vi "blink led.vi"() -> ()   [LabVIEW 2020]
panel:
  in  "stop":bool
  out "Boolean":bool
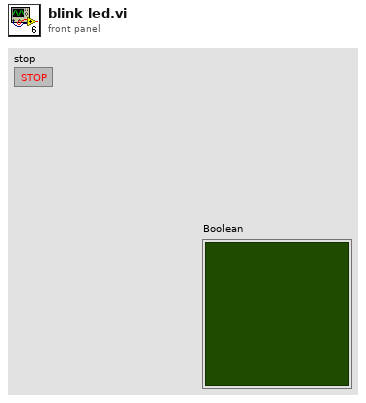
[diagram p1: front panel]
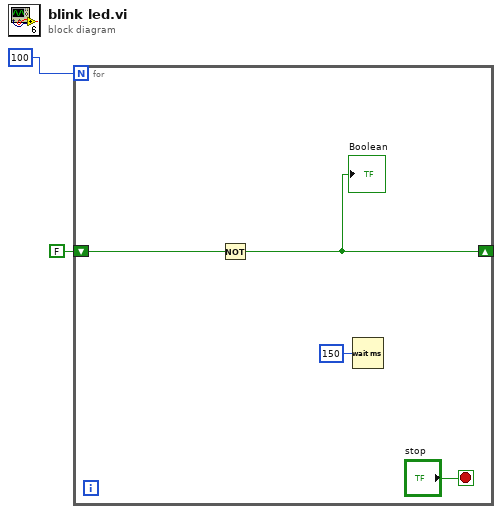
[diagram p0: block diagram]
diagram:
  n1 = for {
    N: 100 -> [_]
    shift-right: [w4] -> _
    shift-left: FALSE -> [w5]
    stop <- "stop" stop-if-true
    n2 = Not(x=w5) -> (.not. x?=w4:bool)
    "Boolean" <- w4
    n3 = Wait (ms)(milliseconds to wait=u32 150) -> ()  [unwired: 1 out]
  }
